vi "Delete Control Point.vi"(0 "FSM.Edge In":refnum<class "FSM.Edge.lvclass">) -> (4 "FSM.Edge Out":refnum<class "FSM.Edge.lvclass">)   [LabVIEW 2020, in "FSM.Edge.lvclass"]
uses:
  FSM.Edge.lvclass
  FSM.Edge.lvclass/FSM.Edge.ctl
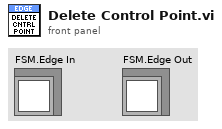
[diagram p1: front panel]
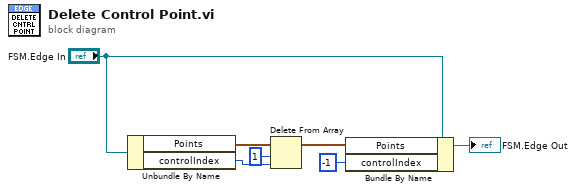
[diagram p0: block diagram]
diagram:
  n1 = Unbundle By Name("FSM.Edge In") -> ("Points"=w5:cluster{"x":i16, "y":i16}[], "controlIndex"=w4:i32)
  n2 = Delete From Array(array=w5, length=1, index=w4) -> (array with subset deleted=w3:cluster{"x":i16, "y":i16}[])  [unwired: 1 out]
  n3 = Bundle By Name(cluster="FSM.Edge In", "Points"=w3, "controlIndex"=-1) -> (→"FSM.Edge Out":refnum<class "FSM.Edge.lvclass">)
